vi "Parse TSA Report File.vi"(8 "error in (no error)":errorcluster, 11 "TSA Report File Path":path) -> (0 "error out":errorcluster, 3 "TSA Messages[]":T1[](array[typedef]))   [LabVIEW 2014, in "SLL TestStand.lvlib"]
uses:
  SLL TestStand.lvlib
  _Typedefs/TSA Message Cluster.ctl
  SLL File IO/XML/_SubVIs/Initialize XML from File.vi
  SLL File IO/XML/_SubVIs/Get XPath Text.vi
  SLL File IO/SLL File IO.lvlib
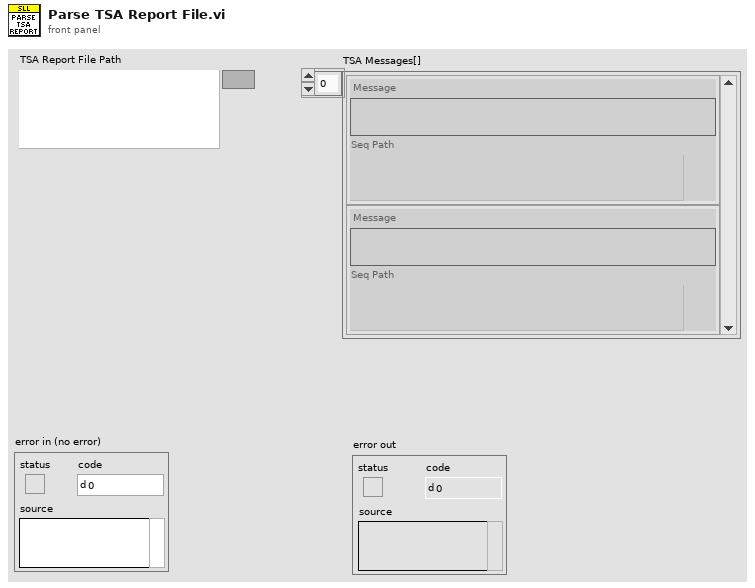
[diagram p1: front panel]
types:
  T1 = typedef "SLL TestStand.lvlib/TSA Message Cluster.ctl" = cluster{"Message":string, "Seq Path":path}
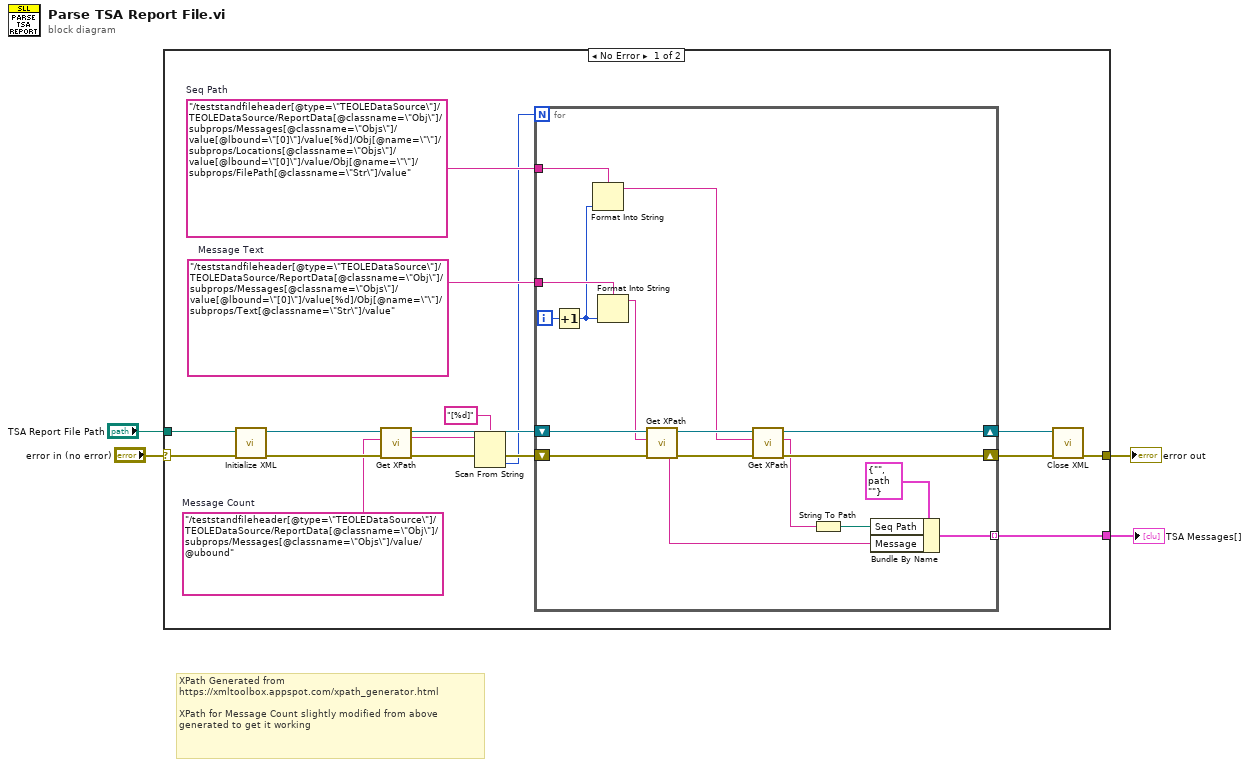
[diagram p0: block diagram]
diagram:
  # "XPath Generated from\nhttps://xmltoolbox.appspot.com/xpath_generator.html\n\nXPath for Message Count slightly modified from above generated to get it working"
  n1 = case shown="No Error" "error in (no error)" {
    selector: "error in (no error)" -> [w21 w39]
    tunnel: [w11 w39] -> w3
    tunnel: "TSA Report File Path" -> [w19 _]
    tunnel: [w9 _] -> w1
    frame No Error {
      w12 = "/teststandfileheader[@type=\"TEOLEDataSource\"]/TEOLEDataSource/ReportData[@classname=\"Obj\"]/subprops/Messages[@classname=\"Objs\"]/value[@lbound=\"[0]\"]/value[%d]/Obj[@name=\"\"]/subprops/Locations[@classname=\"Objs\"]/value[@lbound=\"[0]\"]/value/Obj[@name=\"\"]/subprops/FilePath[@classname=\"Str\"]/value"  # Seq Path
      w13 = "/teststandfileheader[@type=\"TEOLEDataSource\"]/TEOLEDataSource/ReportData[@classname=\"Obj\"]/subprops/Messages[@classname=\"Objs\"]/value[@lbound=\"[0]\"]/value[%d]/Obj[@name=\"\"]/subprops/Text[@classname=\"Str\"]/value"  # Message Text
      w16 = "/teststandfileheader[@type=\"TEOLEDataSource\"]/TEOLEDataSource/ReportData[@classname=\"Obj\"]/subprops/Messages[@classname=\"Objs\"]/value/@ubound"  # Message Count
      n2 = call-poly "Initialize XML.vi"("error in (no error)"=w21, "XML File Path"=w19) -> ("error out"=w20:errorcluster, "DOM document out"=w17:refnum<k20>)  [unwired: 8 in]
      n3 = call-poly "Get XPath.vi"("error in (no error)"=w20, "XPath Expression"=w16, "DOM document in"=w17) -> ("error out"=w18:errorcluster, "Node Text"=w7:string, "DOM document out"=w14:refnum<k20>)  [unwired: 6 in]
      n4 = Scan From String(format string="[%d]", input string=w7, error in=w18) -> (error out=w8:errorcluster, output 1=w5:i32)  [unwired: 2 in, 2 out]
      n5 = for {
        N: w5 -> [_]
        shift-right: [w31] -> w15
        shift-left: w8 -> [w38]
        shift-right: [w29] -> w10
        shift-left: w14 -> [w36]
        tunnel: w13 -> [w35]
        tunnel: w12 -> [w34]
        tunnel: [w23] -> w9 mode=indexing
        i -> [w33]
        n6 = Increment(x=w33) -> (x+1=w22:i32)
        n7 = Format Into String(format string=w34, w22) -> (resulting string=w28:string)  [unwired: 2 in, 1 out]
        n8 = Format Into String(format string=w35, w22) -> (resulting string=w32:string)  [unwired: 2 in, 1 out]
        n9 = call-poly "Get XPath.vi"("error in (no error)"=w38, "XPath Expression"=w32, "DOM document in"=w36) -> ("error out"=w37:errorcluster, "Node Text"=w24:string, "DOM document out"=w30:refnum<k20>)  [unwired: 6 in]
        n10 = call-poly "Get XPath.vi"("error in (no error)"=w37, "XPath Expression"=w28, "DOM document in"=w30) -> ("error out"=w31:errorcluster, "Node Text"=w26:string, "DOM document out"=w29:refnum<k20>)  [unwired: 6 in]
        n11 = String To Path(string=w26) -> (path=w25:path)
        n12 = Bundle By Name(cluster=T1 {"Message"="", "Seq Path"=path ""} ("TSA Message"), "Seq Path"=w25, "Message"=w24) -> (w23:T1)
      }
      n13 = call "Close XML.vi"("error in (no error)"=w15, "DOM document in"=w10) -> ("error out"=w11:errorcluster)  [unwired: 9 in]
    }
    frame Error {
    }
  }
  "error out" <- w3
  "TSA Messages[]" <- w1
